vi "Linear and Log Graph.vi"() -> ()   [LabVIEW 2015]
panel:
  out "Logrithmic":dbl[](array[numeric])
  in  "Max 2":dbl
  in  "Min 2":dbl
  in  "Number of Elements 2":i32
  out "Waveform Graph":dbl[][](graph)
  out "Linear":dbl[](array[numeric])
  in  "Number of Elements":i32
  in  "Min":dbl
  in  "Max":dbl
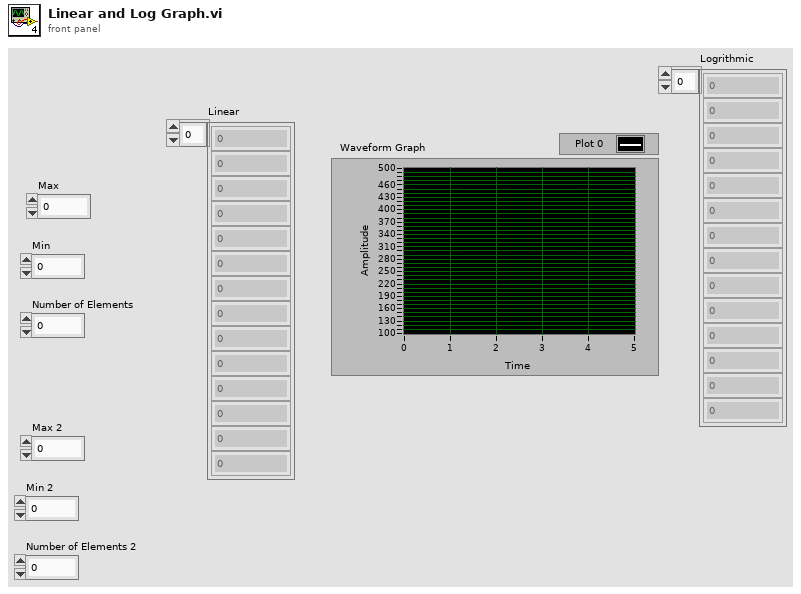
[diagram p1: front panel]
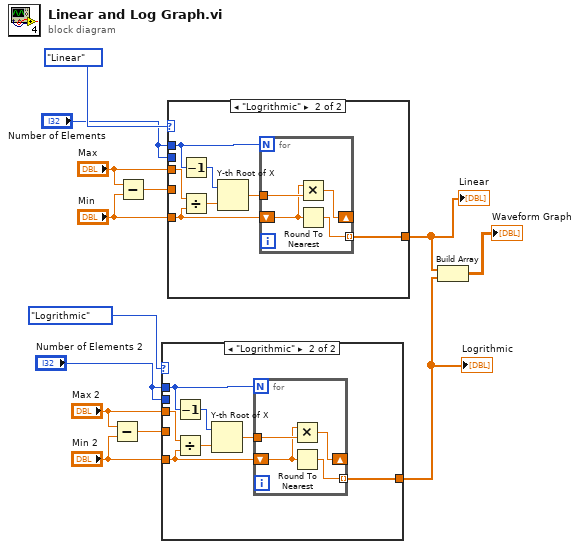
[diagram p0: block diagram]
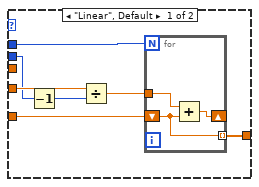
[diagram p2: hidden frame]
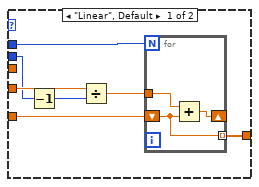
[diagram p3: hidden frame]
diagram:
  n1 = Subtract(x="Max 2", y="Min 2") -> (x-y=w4:dbl)
  n2 = Subtract(x="Max", y="Min") -> (x-y=w13:dbl)
  n3 = case shown="\"Logrithmic\"" enum16{"Linear", "Logrithmic"}."Logrithmic" ("Enum 2") {
    tunnel: w4 -> [w19 _]
    tunnel: "Min 2" -> [w18 w25]
    tunnel: [w17 w28] -> w1
    tunnel: "Number of Elements 2" -> [w16 w27]
    tunnel: "Max 2" -> [_ w26]
    tunnel: "Number of Elements 2" -> [w15 _]
    frame "Linear", Default {
      n4 = Decrement(x=w15) -> (x-1=w14:i32)
      n5 = Divide(x=w19, y=w14) -> (x/y=w20:dbl)
      n6 = for {
        N: w16 -> [_]
        tunnel: w20 -> [w23]
        tunnel: [w22] -> w17 mode=indexing
        shift-right: [w21] -> _
        shift-left: w18 -> [w22]
        n7 = Add(x=w23, y=w22) -> (x+y=w21:dbl)
      }
    }
    frame "Logrithmic" {
      n8 = Decrement(x=w27) -> (x-1=w24:i32)
      n9 = Divide(x=w26, y=w25) -> (x/y=w29:dbl)
      n10 = Y-th Root of X(1:w29, 2:w24) -> (0:w30:dbl)
      n11 = for {
        N: w27 -> [_]
        tunnel: w30 -> [w34]
        tunnel: [w31] -> w28 mode=indexing
        shift-right: [w33] -> _
        shift-left: w25 -> [w32]
        n12 = Multiply(x=w32, y=w34) -> (x*y=w33:dbl)
        n13 = Round To Nearest(number=w32) -> (nearest integer value=w31:dbl)
      }
    }
  }
  "Logrithmic" <- w1
  n14 = case shown="\"Logrithmic\"" enum16{"Linear", "Logrithmic"}."Linear" ("Enum") {
    tunnel: w13 -> [w40 _]
    tunnel: "Min" -> [w39 w46]
    tunnel: [w38 w49] -> w2
    tunnel: "Number of Elements" -> [w37 w48]
    tunnel: "Max" -> [_ w47]
    tunnel: "Number of Elements" -> [w36 _]
    frame "Linear", Default {
      n15 = Decrement(x=w36) -> (x-1=w35:i32)
      n16 = Divide(x=w40, y=w35) -> (x/y=w41:dbl)
      n17 = for {
        N: w37 -> [_]
        tunnel: w41 -> [w44]
        tunnel: [w43] -> w38 mode=indexing
        shift-right: [w42] -> _
        shift-left: w39 -> [w43]
        n18 = Add(x=w44, y=w43) -> (x+y=w42:dbl)
      }
    }
    frame "Logrithmic" {
      n19 = Decrement(x=w48) -> (x-1=w45:i32)
      n20 = Divide(x=w47, y=w46) -> (x/y=w50:dbl)
      n21 = Y-th Root of X(1:w50, 2:w45) -> (0:w51:dbl)
      n22 = for {
        N: w48 -> [_]
        tunnel: w51 -> [w55]
        tunnel: [w52] -> w49 mode=indexing
        shift-right: [w54] -> _
        shift-left: w46 -> [w53]
        n23 = Multiply(x=w53, y=w55) -> (x*y=w54:dbl)
        n24 = Round To Nearest(number=w53) -> (nearest integer value=w52:dbl)
      }
    }
  }
  "Linear" <- w2
  n25 = Build Array(w2, w1) -> (→"Waveform Graph":dbl[][])
